vi "LcWebView_example_1.vi"() -> ()   [LabVIEW 2020, in "LcWebView.lvclass"]
uses:
  LcWebView.lvclass
  C:/Projects/WebView2/LcWebView/data/Microsoft.Web.WebView2.WinForms.dll
  data/Microsoft.Web.WebView2.WinForms.dll
panel:
  out "Loaded":bool
  out "Javascript result":string
  out "DocumentTitle":string
  out "HTML content":string
  out "Initialise Loops":i32
  out "Status Message":string
  out "Status":i32(ring) items=["Created", "WaitingForActivation", "WaitingToRun", "Running", "WaitingForChildrenToComplete", "RanToCompletion", "Canceled", "Faulted"]
  out "Error Out":errorcluster
  in  "stop":bool
  in  "Web":refnum<k24>(container)
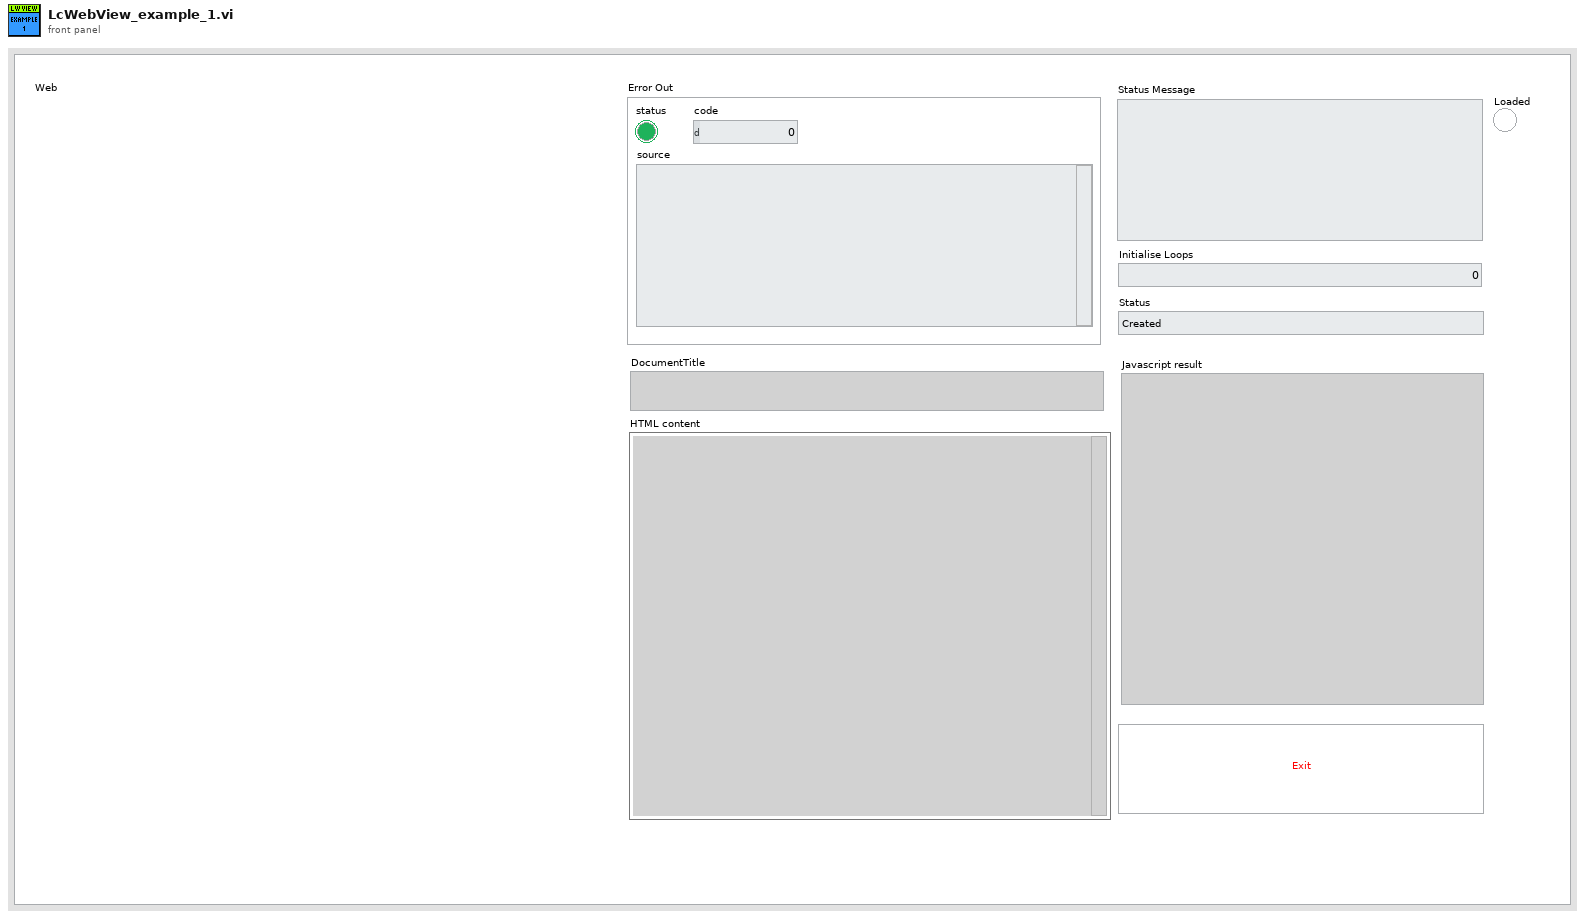
[diagram p1: front panel]
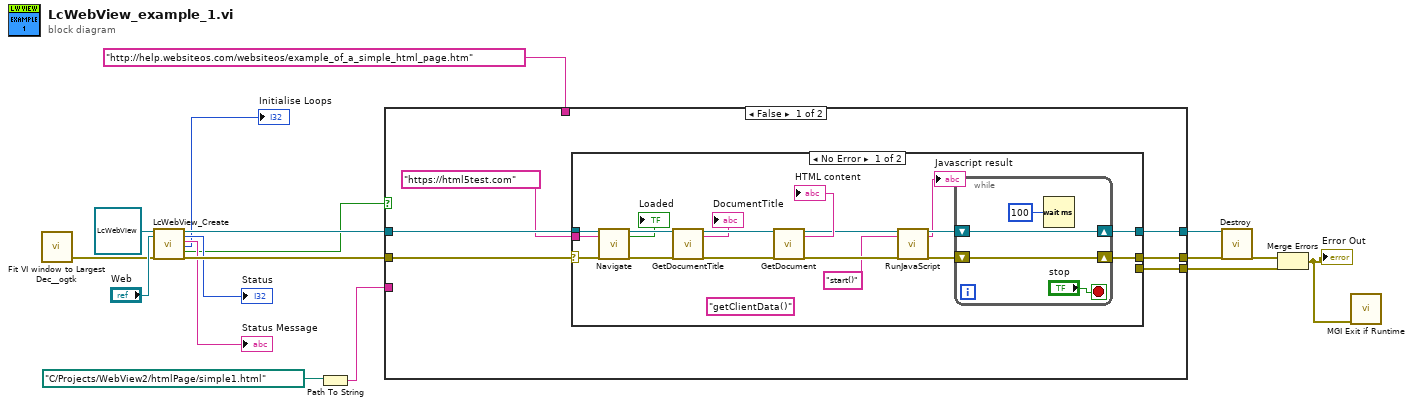
[diagram p0: block diagram]
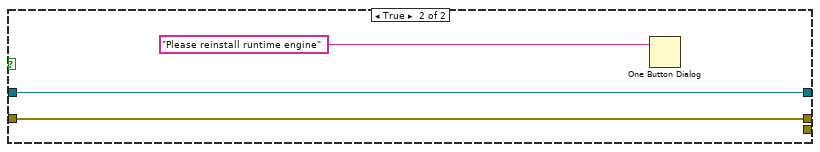
[diagram p3: hidden frame]
diagram:
  n1 = call <userlib>:"Fit VI window to Largest Dec__ogtk.vi"() -> ("error out"=w2:errorcluster)  [unwired: 6 in, 1 out]
  n2 = call "LcWebView_Create.vi"("reference in"=refnum<class "LcWebView.lvclass"> refnum, "Webview container"="Web", "Error In"=w2) -> ("reference out"=w15:refnum<class "LcWebView.lvclass">, "Status"=→"Status":i32, "Status Message"=→"Status Message":string, "Initialise Loops"=→"Initialise Loops":i32, "Reinstall Runtime"=w3:bool, "Error Out"=w14:errorcluster)  [unwired: 9 in, 2 out]
  n3 = Path To String(path=path "C:/Projects/WebView2/htmlPage/simple1.html" ("DLLs path In")) -> (string=w4:string)
  n4 = case shown="False" w3 {
    tunnel: w15 -> [w23 w50]
    tunnel: w14 -> [w22 w49]
    tunnel: [w21 w50] -> w13
    tunnel: [w20 w49] -> w12
    tunnel: [w19 _] -> w7
    tunnel: "http://help.websiteos.com/websiteos/example_of_a_simple_html_page.htm" ("URL") -> [_ _]
    tunnel: w4 -> [_ _]
    frame False {
      n5 = case shown="No Error" w22 {
        selector: w22 -> [w40 w46]
        tunnel: w23 -> [w41 w47]
        tunnel: [w39 w47] -> w21
        tunnel: [w38 _] -> w20
        tunnel: [_ w46] -> w19
        tunnel: "https://html5test.com" ("URL") -> [w31 _]
        frame No Error {
          (unwired) "getClientData()" ("Java Script Function")
          n6 = call-dynamic "Navigate.vi"("reference in"=w41, "URL"=w31, "Error In"=w40) -> ("reference out"=w36:refnum<class "LcWebView.lvclass">, "Loaded"=→"Loaded":bool, "Error Out"=w35:errorcluster)  [unwired: 14 in]
          n7 = call-dynamic "GetDocumentTitle.vi"("reference in"=w36, "Error In"=w35) -> ("reference out"=w34:refnum<class "LcWebView.lvclass">, "DocumentTitle"=→"DocumentTitle":string, "Error Out"=w33:errorcluster)  [unwired: 15 in]
          n8 = call-dynamic "GetDocument.vi"("reference in"=w34, "Error In"=w33) -> ("reference out"=w30:refnum<class "LcWebView.lvclass">, "Result"=→"HTML content":string, "Error Out"=w29:errorcluster)  [unwired: 15 in]
          n9 = call-dynamic "RunJavaScript.vi"("reference in"=w30, "Java Script Function"="start()", "Error In"=w29) -> ("reference out"=w28:refnum<class "LcWebView.lvclass">, "Result"=→"Javascript result":string, "Error Out"=w27:errorcluster)  [unwired: 13 in, 1 out]
          n10 = while {
            shift-right: [w44] -> w39
            shift-left: w28 -> [w44]
            shift-right: [w43] -> w38
            shift-left: w27 -> [w43]
            stop <- "stop" stop-if-true
            n11 = Wait (ms)(milliseconds to wait=u32 100) -> ()  [unwired: 1 out]
          }
        }
        frame Error {
        }
      }
    }
    frame True {
      n12 = One Button Dialog(message="Please reinstall runtime engine") -> ()  [unwired: 1 in, 1 out]
    }
  }
  n13 = call-dynamic "Destroy.vi"("reference in"=w13, "Error In"=w12) -> ("Error Out"=w11:errorcluster)  [unwired: 16 in, 1 out]
  n14 = Merge Errors(w11, w7) -> (w1:errorcluster)
  "Error Out" <- w1
  n15 = call <userlib>:"MGI Exit if Runtime.vi"("Error In (Dependency Only)"=w1) -> ()  [unwired: 11 in]
